vi "_BlankServer.vi"() -> ()   [LabVIEW 2012]
uses:
  <userlib>/ROSforLV/ROS/Code/SubVIs/_ROSControl.ctl
  <userlib>/ROSforLV/ROS/Code/SubVIs/_ROSDirection.ctl
  <userlib>/ROSforLV/ROS/Code/Console/Servers/ServerSubs/ROSLog.ctl
  <userlib>/ROSforLV/ROS/Code/Console/Servers/ServerSubs/MyState.ctl
  <userlib>/ROSforLV/ROS/Code/Console/Servers/ServerSubs/requestTopic.ctl
panel:
  out "Log of port":string
  out "Queue log":string
  out "Last Reply":string
  out "Registered topics":T1[](array[typedef])
  out "Registering":bool
  out "MyState":T3
  out "Setup":string
  out "Cmd Log":T4[](array[typedef])
  out "Connections":T5(array[cluster])
  in  "stop":bool
  in  "ROS":T1={"topic port"=1236, "Node"="/labview", "topic"="/robot/head/command_head_nod", "type"="std_msgs/Bool", "node port"=7000, "error "={"status"=FALSE, "code"=0, "source"=""}, "Direction"=enum."Publisher", "APIs"=[], "Update (ms)"=1, "write queue"=1}
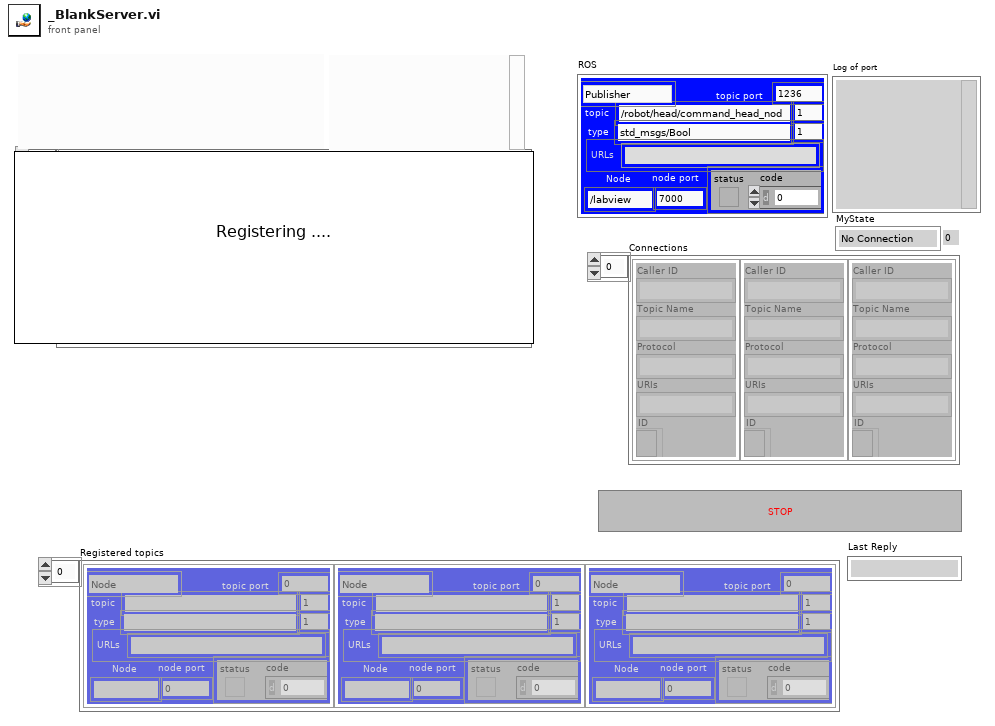
[diagram p1: front panel]
types:
  T1 = typedef "_ROSControl.ctl" = cluster{"topic port":u16, "Node":string, "topic":string, "type":string, "node port":u32, "error ":errorcluster, "Direction":T2, "APIs":string[], "Update (ms)":u16, "write queue":u16}
  T2 = typedef "_ROSDirection.ctl" = enum16{"Node", "Publisher", "Subscriber", "Service Client"}
  T3 = typedef "MyState.ctl" = enum16{"No Connection", "Registered", "Connected", "Close"}
  T4 = typedef "ROSLog.ctl" = cluster{"Sent":string, "Reply":string, "MethodName":string, "success":bool, "Dir1":string, "Dir2":string, "Time Stamp":string, "error":errorcluster, "Preamble":string}
  T5 = cluster{"Caller ID":string, "Topic Name":string, "Protocol":string, "URIs":string, "ID":refnum<k5>}[]
  T6 = enum16{"Reset Log", "Add Client", "Remove Client", "Add Task"}
  T7 = typedef "requestTopic.ctl" = cluster{"New Subscriber":cluster{"Caller ID":string, "Topic Name":string, "Protocol":string, "URIs":string, "ID":refnum<k5>}, "ROS of Server":T1, "new port":u16}
  T8 = cluster{"Code":i32, "Status Message":string, "APIs":string[]}
  T9 = cluster{"Caller ID":string, "Topic Name":string, "Protocol":string, "URIs":string, "ID":refnum<k5>}
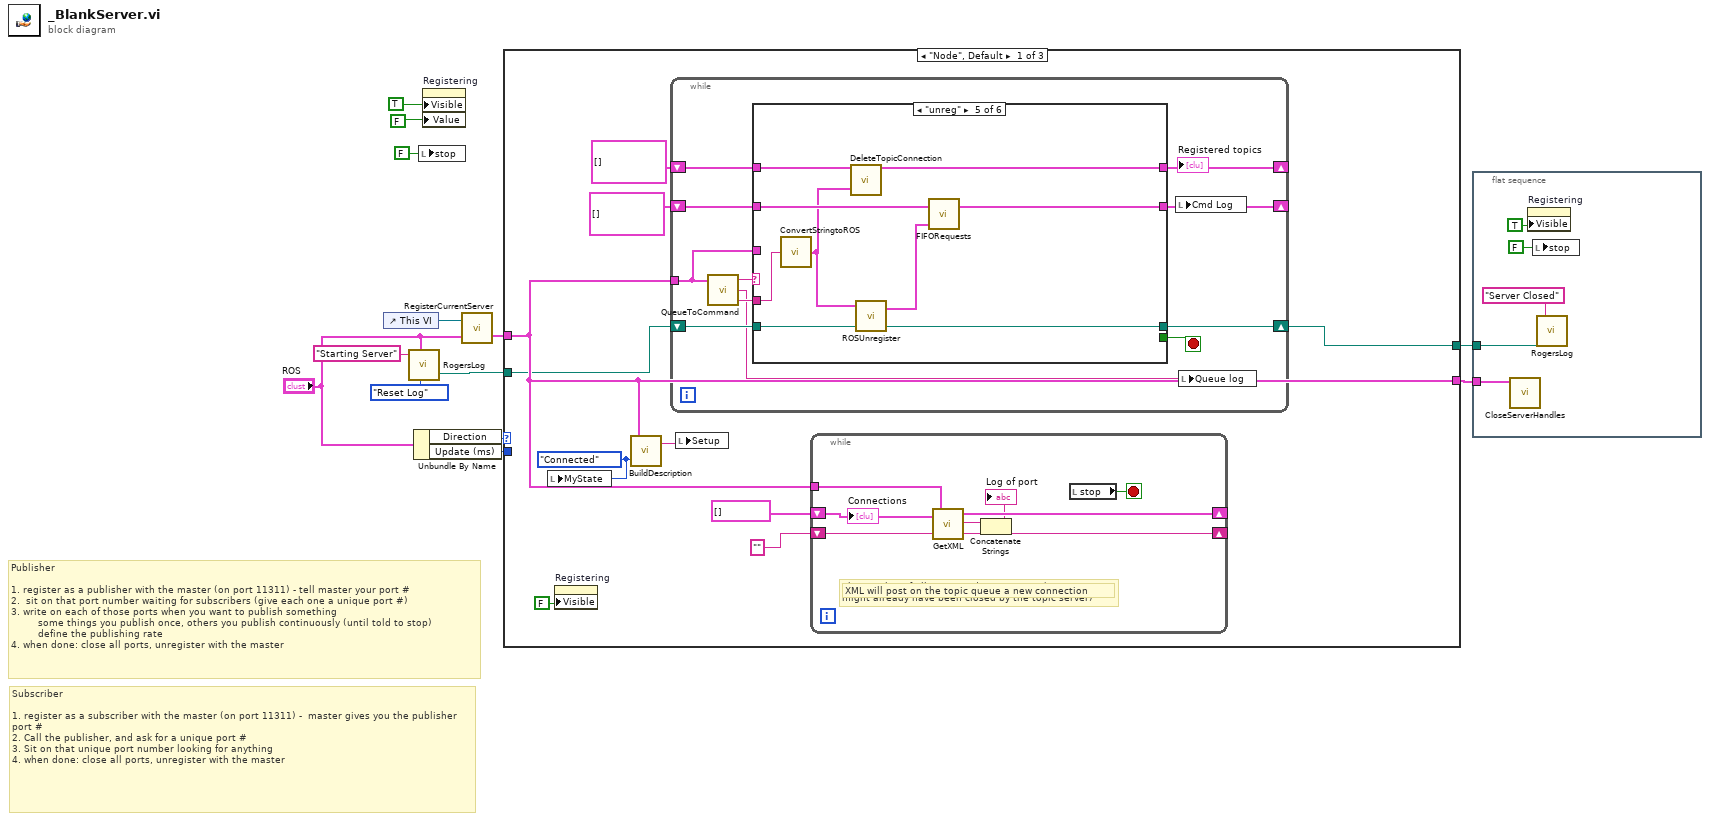
[diagram p0: block diagram]
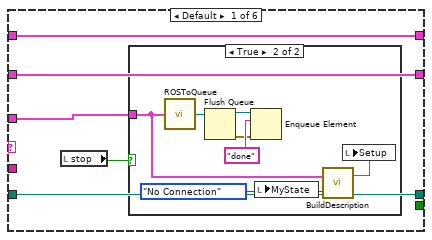
[diagram p2: hidden frame]
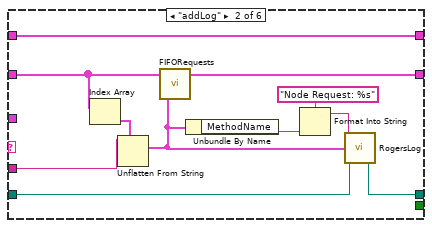
[diagram p4: hidden frame]
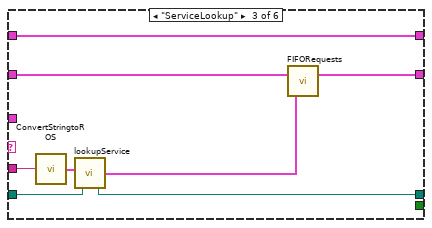
[diagram p5: hidden frame]
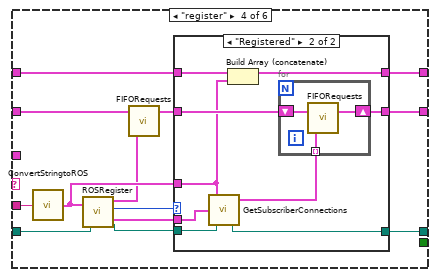
[diagram p6: hidden frame]
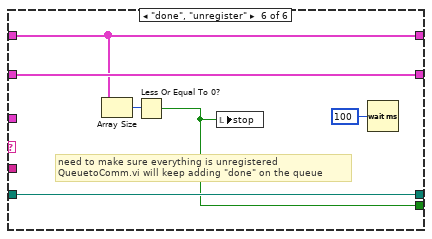
[diagram p8: hidden frame]
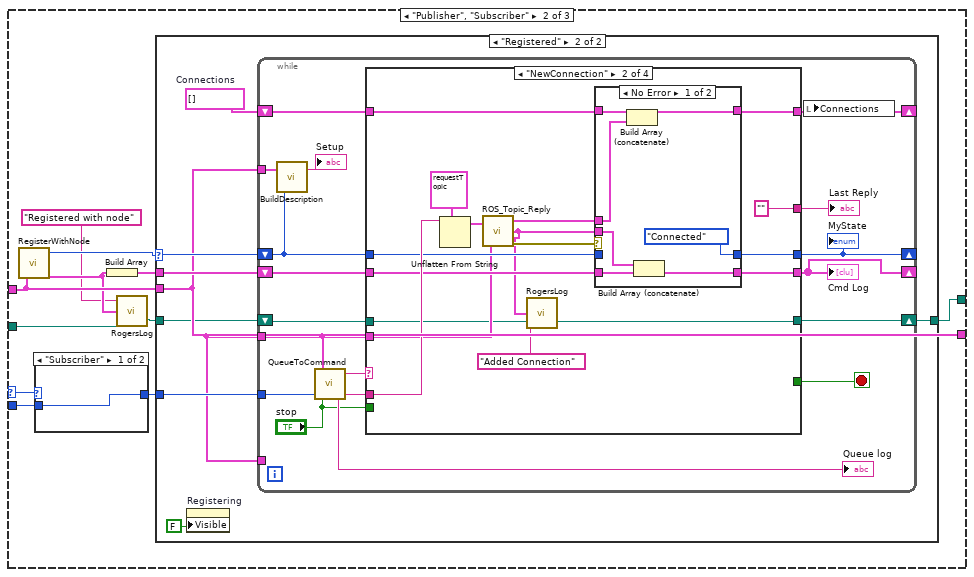
[diagram p9: hidden frame]
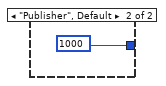
[diagram p10: hidden frame]
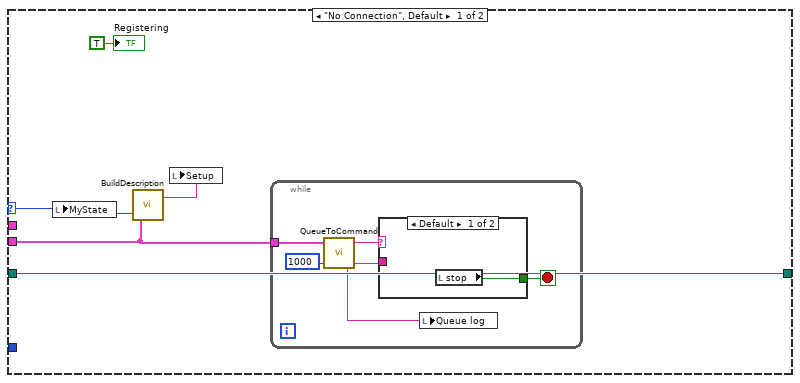
[diagram p11: hidden frame]
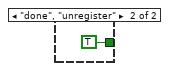
[diagram p12: hidden frame]
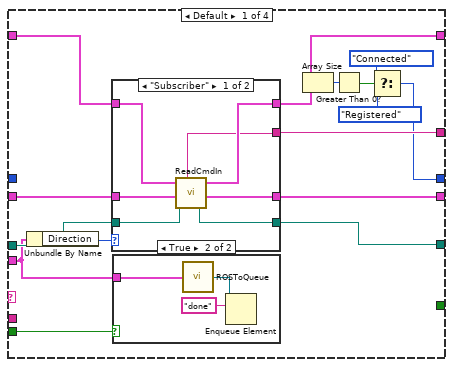
[diagram p13: hidden frame]
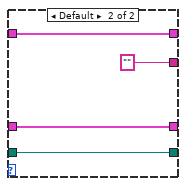
[diagram p14: hidden frame]
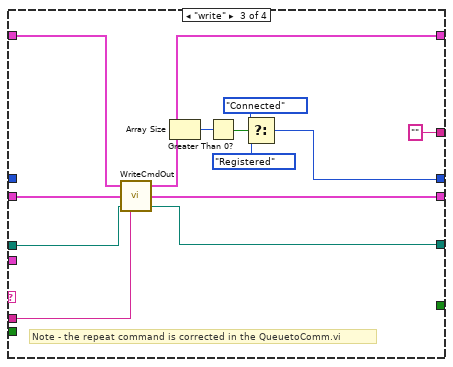
[diagram p17: hidden frame]
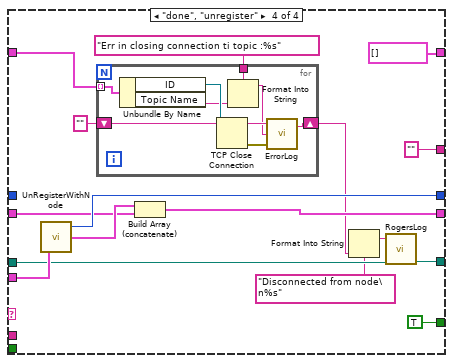
[diagram p18: hidden frame]
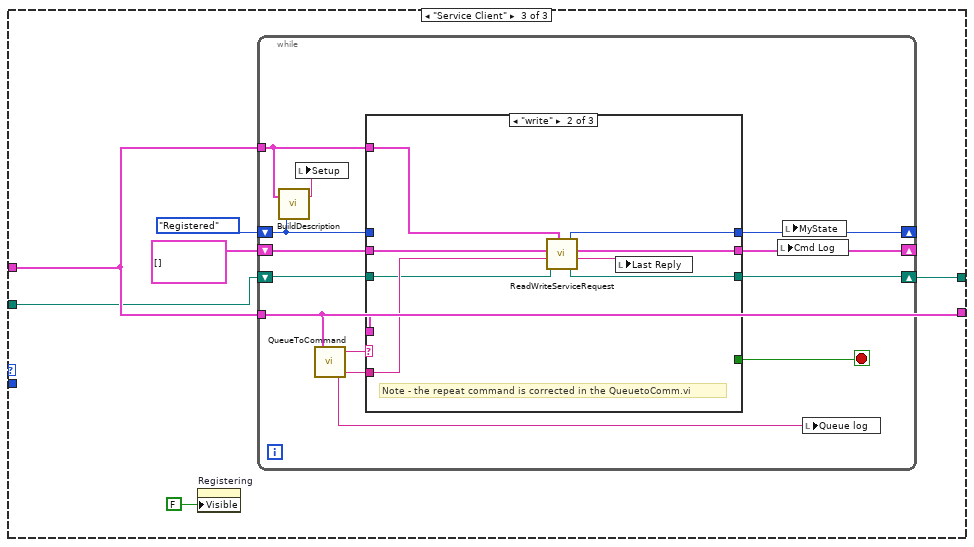
[diagram p19: hidden frame]
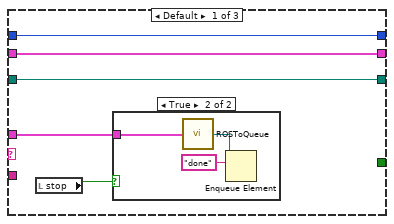
[diagram p20: hidden frame]
diagram:
  # "Subscriber\n\n1. register as a subscriber with the master (on port 11311) -  master gives you the publisher port #\n2. Call the publisher, and ask for a unique port #\n3. Sit on that unique port number looking for anything\n4. when done: close all ports, unregister with the master"
  # "Publisher\n\n1. register as a publisher with the master (on port 11311) - tell master your port #\n2.  sit on that port number waiting for subscribers (give each one a unique port #)\n3. write on each of those ports when you want to publish something\n         some things you publish once, others you publish continuously (until told to stop)\n         define the publishing rate\n4. when done: close all ports, unregister with the master"
  n1 = control-ref of="This VI"() -> (w8:refnum<vi>)
  n2 = call <userlib>:"RogersLog.vi"("Text to add"="Starting Server", "ROS"="ROS", "Task"=T6."Reset Log") -> ("LogPath out"=w2:path)  [unwired: 2 in, 1 out]
  n3 = Unbundle By Name("ROS") -> ("Direction"=w11:T2, "Update (ms)"=w6:u16)
  n4 = local write "stop"(FALSE ("stop")) -> ()
  n5 = property on="Registering" class="Bool (strict)"("Visible"=TRUE ("Registering"), "Value"=FALSE ("Registering")) -> ()  [unwired: 2 in, 2 out]
  n6 = call <userlib>:"RegisterCurrentServer.vi"("ROS in"="ROS", "This VI"=w8) -> ("ROS out"=w7:T1)  [unwired: 1 in]
  n7 = case shown="\"Node\", Default" w11 {
    selector: w11 -> [_ w124 _]
    tunnel: w7 -> [w18 w126 w266]
    tunnel: [w18 w126 w266] -> w9
    tunnel: w6 -> [_ w121 _]
    tunnel: w2 -> [w15 w120 w262]
    tunnel: [w14 w118 w261] -> w1
    frame "Node", Default {
      w21 = MyState."Connected" ("MyState")
      n8 = local write "MyState"(w21) -> ()
      n9 = property on="Registering" class="Bool (strict)"("Visible"=FALSE ("Registering")) -> ()  [unwired: 2 in, 2 out]
      n10 = call <userlib>:"BuildDescription.vi"("MyState"=w21, "ROS in"=w18) -> ("Setup"=w22:string)  [unwired: 1 in]
      n11 = while {
        shift-right: [w25] -> w14
        shift-left: w15 -> [w33]
        shift-right: [w26] -> _
        shift-left: T4[] [] ("Requests Out") -> [w32]
        shift-right: [w31] -> _
        shift-left: T1[] [] -> [w30]
        tunnel: w18 -> [w24]
        stop <- w34 stop-if-true
        n12 = call <userlib>:"QueueToCommand.vi"("ROS"=w24) -> ("data"=w28:string, "Queue log"=w27:string, "Command"=w29:string)  [unwired: 2 in]
        n13 = case shown="\"unreg\"" w29 {
          tunnel: [_ _ _ _ _ w104] -> w34
          tunnel: w28 -> [_ w56 w64 w78 w102 _]
          tunnel: w33 -> [w39 w48 w59 w77 w101 w108]
          tunnel: [w39 w47 w58 w66 w100 w108] -> w25
          tunnel: [w38 w53 w60 w76 w98 w107] -> w26
          tunnel: w32 -> [w38 w54 w61 w69 w99 w107]
          tunnel: [w37 w57 w65 w74 w95 w106] -> w31
          tunnel: w30 -> [w37 w57 w65 w75 w96 w106]
          tunnel: w24 -> [w35 _ _ _ _ _]
          frame Default {
            n14 = local read "stop"() -> (w36:bool)
            n15 = case shown="True" w36 {
              tunnel: w35 -> [_ w41]
              frame False {
              }
              frame True {
                w42 = MyState."No Connection" ("MyState")
                n16 = call <userlib>:"ROSToQueue.vi"("ROS"=w41) -> ("queue"=w44:refnum<queue>)  [unwired: 3 in, 1 out]
                n17 = Flush Queue(queue=w44) -> (queue out=w40:refnum<queue>, error out=w45:errorcluster)  [unwired: 1 in, 1 out]
                n18 = Enqueue Element(queue=w40, element="done" ("regular expression"), error in (no error)=w45) -> ()  [unwired: 1 in, 3 out]
                n19 = local write "MyState"(w42) -> ()
                n20 = call <userlib>:"BuildDescription.vi"("MyState"=w42, "ROS in"=w41) -> ("Setup"=w43:string)  [unwired: 1 in]
                n21 = local write "Setup"(w43) -> ()
              }
            }
          }
          frame "addLog" {
            n22 = Index Array(array=w54) -> (element=w55:T4)  [unwired: 1 in]
            n23 = Unflatten From String(type=w55, binary string=w56) -> (value=w51:T4)  [unwired: 3 in, 2 out]
            n24 = call <userlib>:"FIFORequests.vi"("Log"=w51, "Requests in"=w54) -> ("Requests out"=w53:T4[])  [unwired: 1 in]
            n25 = Unbundle By Name(w51) -> ("MethodName"=w50:string)
            n26 = Format Into String(format string="Node Request: %s", w50) -> (resulting string=w49:string)  [unwired: 2 in, 1 out]
            n27 = call <userlib>:"RogersLog.vi"("Text to add"=w49, "Log"=w51, "LogPath in"=w48) -> ("LogPath out"=w47:path)  [unwired: 2 in, 1 out]
          }
          frame "ServiceLookup" {
            n28 = call <userlib>:"ConvertStringtoROS.vi"("string in"=w64) -> ("ROS"=w63:T1)
            n29 = call <userlib>:"lookupService.vi"("Err In"=w59, "Service ROS"=w63) -> ("Err Out"=w58:path, "Log"=w62:T4)  [unwired: 2 in]
            n30 = call <userlib>:"FIFORequests.vi"("Log"=w62, "Requests in"=w61) -> ("Requests out"=w60:T4[])  [unwired: 1 in]
          }
          frame "register" {
            n31 = call <userlib>:"ConvertStringtoROS.vi"("string in"=w78) -> ("ROS"=w73:T1)
            n32 = call <userlib>:"ROSRegister.vi"("Err In"=w77, "ROS to register"=w73) -> ("Err Out"=w67:path, "Response"=w72:T8, "MyState"=w71:T3, "Log"=w70:T4)
            n33 = call <userlib>:"FIFORequests.vi"("Log"=w70, "Requests in"=w69) -> ("Requests out"=w68:T4[])  [unwired: 1 in]
            n34 = case shown="\"Registered\"" w71 {
              tunnel: w68 -> [w80 w90]
              tunnel: [w80 w89] -> w76
              tunnel: w75 -> [w81 w88]
              tunnel: [w81 w87] -> w74
              tunnel: w73 -> [_ w85]
              tunnel: w72 -> [_ w84]
              tunnel: w67 -> [w79 w83]
              tunnel: [w79 w82] -> w66
              frame Default {
              }
              frame "Registered" {
                n35 = call <userlib>:"GetSubscriberConnections.vi"("Err in"=w83, "Response"=w84, "ROS registered"=w85) -> ("Err out"=w82:path, "Logs out"=w86:T4[])  [unwired: 1 out]
                n36 = Build Array (concatenate)(w88, w85) -> (w87:T1[])
                n37 = for {
                  tunnel: w86 -> [w91] mode=indexing
                  shift-right: [w92] -> w89
                  shift-left: w90 -> [w93]
                  n38 = call <userlib>:"FIFORequests.vi"("Log"=w91, "Requests in"=w93) -> ("Requests out"=w92:T4[])  [unwired: 1 in]
                }
              }
            }
          }
          frame "unreg" {
            n39 = call <userlib>:"ConvertStringtoROS.vi"("string in"=w102) -> ("ROS"=w94:T1)
            n40 = call <userlib>:"DeleteTopicConnection.vi"("ROS"=w94, "Con In"=w96) -> ("Con out"=w95:T1[])
            n41 = call <userlib>:"ROSUnregister.vi"("Err in"=w101, "Server ROS"=w94) -> ("Err out"=w100:path, "Log"=w97:T4)  [unwired: 1 in]
            n42 = call <userlib>:"FIFORequests.vi"("Log"=w97, "Requests in"=w99) -> ("Requests out"=w98:T4[])  [unwired: 1 in]
          }
          frame "done", "unregister" {
            # "need to make sure everything is unregistered\nQueuetoComm.vi will keep adding \"done\" on the queue"
            n43 = Array Size(array=w106) -> (size(s)=w105:i32)
            n44 = Less Or Equal To 0?(x=w105) -> (x <= 0?=w104:bool)
            n45 = local write "stop"(w104) -> ()
            n46 = Wait (ms)(milliseconds to wait=u32 100) -> ()  [unwired: 1 out]
          }
        }
        "Registered topics" <- w31
        n47 = local write "Cmd Log"(w26) -> ()
        n48 = local write "Queue log"(w27) -> ()
      }
      n49 = local write "Setup"(w22) -> ()
      n50 = while {
        shift-right: [w115] -> _
        shift-left: T5 [] ("Subscribers") -> [w109]
        tunnel: w18 -> [w114]
        shift-right: [w110] -> _
        shift-left: "" ("String out") -> [w112]
        stop <- w113 stop-if-true
        # "This is a log of all requested connections (some\nmight already have been closed by the topic server)"
        # "XML will post on the topic queue a new connection"
        n51 = call <userlib>:"GetXML.vi"("Node ROS"=w114, "Subscribers in"=w109) -> ("reply"=w111:string, "Subscribers Out"=w115:T5)  [unwired: 1 in]
        n52 = Concatenate Strings(w111, w112) -> (w110:string)
        "Log of port" <- w110
        n53 = local read "stop"() -> (w113:bool)
        "Connections" <- w109
      }
    }
    frame "Publisher", "Subscriber" {
      n54 = call <userlib>:"RegisterWithNode.vi"("ROS"=w126) -> ("MyState"=w125:T3, "Log"=w117:T4)  [unwired: 1 in]
      n55 = case shown="\"Subscriber\"" w124 {
        tunnel: [w127 1000 ("timeout in ms (1000)")] -> w123
        tunnel: w121 -> [w127 _]
        frame "Subscriber" {
        }
        frame "Publisher", Default {
        }
      }
      n56 = Build Array(w117) -> (w122:T4[])
      n57 = call <userlib>:"RogersLog.vi"("Text to add"="Registered with node" ("format string"), "Log"=w117, "LogPath in"=w120) -> ("LogPath out"=w119:path)  [unwired: 2 in, 1 out]
      n58 = case shown="\"Registered\"" w125 {
        selector: w125 -> [w132 w148]
        tunnel: w126 -> [w130 w143]
        tunnel: w123 -> [_ w146]
        tunnel: w122 -> [_ w145]
        tunnel: w119 -> [w129 w144]
        tunnel: [w129 w142] -> w118
        frame "No Connection", Default {
          n59 = local write "MyState"(w132) -> ()
          n60 = call <userlib>:"BuildDescription.vi"("MyState"=w132, "ROS in"=w130) -> ("Setup"=w133:string)  [unwired: 1 in]
          n61 = local write "Setup"(w133) -> ()
          n62 = while {
            tunnel: w130 -> [w134]
            stop <- w139 stop-if-true
            n63 = call <userlib>:"QueueToCommand.vi"("timeout"=1000 ("timeout in ms (-1)"), "ROS"=w134) -> ("data"=w138:string, "Queue log"=w135:string, "Command"=w136:string)  [unwired: 1 in]
            n64 = case shown="Default" w136 {
              tunnel: [w140 TRUE] -> w139
              tunnel: w138 -> [_ _]
              frame Default {
                n65 = local read "stop"() -> (w140:bool)
              }
              frame "done", "unregister" {
              }
            }
            n66 = local write "Queue log"(w135) -> ()
          }
          "Registering" <- TRUE ("Registering")
        }
        frame "Registered" {
          w149 = T5 []  # Connections
          n67 = property on="Registering" class="Bool (strict)"("Visible"=FALSE ("Registering")) -> ()  [unwired: 2 in, 2 out]
          n68 = while {
            shift-right: [w150] -> w142
            shift-left: w144 -> [w167]
            shift-right: [w164] -> _
            shift-left: w145 -> [w165]
            shift-right: [w162] -> _
            shift-left: w148 -> [w153]
            tunnel: w143 -> [w161]
            tunnel: w143 -> [w152]
            shift-right: [w155] -> _
            shift-left: w149 -> [w160]
            tunnel: w146 -> [w154]
            tunnel: w143 -> [_]
            stop <- w159 stop-if-true
            n69 = call <userlib>:"BuildDescription.vi"("MyState"=w153, "ROS in"=w161) -> ("Setup"=→"Setup":string)  [unwired: 1 in]
            n70 = call <userlib>:"QueueToCommand.vi"("timeout"=w154, "Stop Btn Pressed?"="stop", "ROS"=w152) -> ("data"=w166:string, "Queue log"=→"Queue log":string, "Command"=w157:string)
            n71 = case shown="\"NewConnection\"" w157 {
              tunnel: [w180 w197 w236 w241] -> w150
              tunnel: w167 -> [w179 w200 w224 w242]
              tunnel: [w171 w204 w227 w252] -> w162
              tunnel: w166 -> [_ w209 w233 _]
              tunnel: w165 -> [w178 w208 w235 w248]
              tunnel: [w181 w207 w234 w247] -> w164
              tunnel: w160 -> [w177 w213 w231 w246]
              tunnel: [w172 w212 w225 T5 [] ("Connections Out")] -> w155
              tunnel: [_ _ _ TRUE] -> w159
              tunnel: [w182 "" ("String out") "" ("String out") "" ("String out")] -> w158
              tunnel: w153 -> [_ w203 _ _]
              tunnel: w152 -> [w169 w201 _ w244]
              tunnel: "stop" -> [w168 _ _ _]
              frame Default {
                n72 = Unbundle By Name(w169) -> ("Direction"=w170:T2)
                n73 = case shown="\"Subscriber\"" w170 {
                  tunnel: [w185 "" ("String out")] -> w182
                  tunnel: [w189 w191] -> w172
                  tunnel: [w188 w192] -> w181
                  tunnel: [w187 w190] -> w180
                  tunnel: w179 -> [w183 w190]
                  tunnel: w178 -> [w186 w192]
                  tunnel: w177 -> [w184 w191]
                  frame "Subscriber" {
                    n74 = call <userlib>:"ReadCmdIn.vi"("Connections"=w184, "Log in"=w186, "Err in"=w183) -> ("data"=w185:string, "Connections out"=w189:T5, "Log out"=w188:T4[], "Err out"=w187:path)  [unwired: 1 in]
                  }
                  frame Default {
                  }
                }
                n75 = case shown="True" w168 {
                  tunnel: w169 -> [_ w194]
                  frame False {
                  }
                  frame True {
                    n76 = call <userlib>:"ROSToQueue.vi"("ROS"=w194) -> ("queue"=w195:refnum<queue>)  [unwired: 3 in, 1 out]
                    n77 = Enqueue Element(queue=w195, element="done") -> ()  [unwired: 2 in, 3 out]
                  }
                }
                n78 = Array Size(array=w172) -> (size(s)=w176:i32)
                n79 = Greater Than 0?(x=w176) -> (x > 0?=w173:bool)
                n80 = Select(t=MyState."Connected" ("f"), s=w173, f=MyState."Registered") -> (s? t:f=w171:T3)
              }
              frame "NewConnection" {
                n81 = Unflatten From String(type=T7 {"New Subscriber"={"Caller ID"="", "Topic Name"="", "Protocol"="", "URIs"="", "ID"=refnum}, "ROS of Server"={"topic port"=0, "Node"="", "topic"="", "type"="", "node port"=0, "error "={"status"=FALSE, "code"=0, "source"=""}, "Direction"=enum."Node", "APIs"=[], "Update (ms)"=0, "write queue"=0}, "new port"=0} ("data"), binary string=w209) -> (value=w206:T7)  [unwired: 3 in, 2 out]
                n82 = call <userlib>:"ROS_Topic_Reply.vi"("data"=w206, "My ROS"=w201) -> ("Subscriber out"=w210:T9, "Log"=w199:T4, "error IO"=w205:errorcluster)
                n83 = call <userlib>:"RogersLog.vi"("Text to add"="Added Connection", "Log"=w199, "LogPath in"=w200) -> ("LogPath out"=w197:path)  [unwired: 2 in, 1 out]
                n84 = case shown="No Error" w205 {
                  tunnel: w213 -> [w220 w223]
                  tunnel: [w219 w223] -> w212
                  tunnel: w210 -> [w218 _]
                  tunnel: w199 -> [w217 _]
                  tunnel: w208 -> [w216 w222]
                  tunnel: [w215 w222] -> w207
                  tunnel: [MyState."Connected" ("MyState") w221] -> w204
                  tunnel: w203 -> [_ w221]
                  frame No Error {
                    n85 = Build Array (concatenate)(w220, w218) -> (w219:T5)
                    n86 = Build Array (concatenate)(w217, w216) -> (w215:T4[])
                  }
                  frame Error {
                  }
                }
              }
              frame "write" {
                # "Note - the repeat command is corrected in the QueuetoComm.vi"
                n87 = call <userlib>:"WriteCmdOut.vi"("Connections In"=w231, "Log in"=w235, "Err in"=w224, "data"=w233) -> ("Connections Out"=w225:T5, "Log out"=w234:T4[], "Err out"=w236:path)  [unwired: 1 in]
                n88 = Array Size(array=w225) -> (size(s)=w226:i32)
                n89 = Greater Than 0?(x=w226) -> (x > 0?=w230:bool)
                n90 = Select(t=MyState."Connected" ("f"), s=w230, f=MyState."Registered") -> (s? t:f=w227:T3)
              }
              frame "done", "unregister" {
                n91 = call <userlib>:"UnRegisterWithNode.vi"("ROS"=w244) -> ("MyState"=w252:T3, "Log"=w249:T4)  [unwired: 2 in]
                n92 = for {
                  tunnel: w246 -> [w260] mode=indexing
                  shift-right: [w258] -> w239
                  shift-left: "" ("String out") -> [w257]
                  tunnel: "Err in closing connection ti topic :%s" ("String in") -> [w255]
                  n93 = Unbundle By Name(w260) -> ("ID"=w259:refnum<k5>, "Topic Name"=w254:string)
                  n94 = TCP Close Connection(connection ID=w259) -> (error out=w256:errorcluster)  [unwired: 2 in, 1 out]
                  n95 = Format Into String(format string=w255, w254) -> (resulting string=w253:string)  [unwired: 2 in, 1 out]
                  n96 = call <userlib>:"ErrorLog.vi"("error in"=w256, "String in"=w253, "Error String"=w257) -> ("String out"=w258:string)  [unwired: 1 out]
                }
                n97 = Build Array (concatenate)(w249, w248) -> (w247:T4[])
                n98 = Format Into String(format string="Disconnected from node\n%s", w239) -> (resulting string=w238:string)  [unwired: 2 in, 1 out]
                n99 = call <userlib>:"RogersLog.vi"("Text to add"=w238, "LogPath in"=w242) -> ("LogPath out"=w241:path)  [unwired: 3 in, 1 out]
              }
            }
            "Cmd Log" <- w164
            "MyState" <- w162
            "Last Reply" <- w158
            n100 = local write "Connections"(w155) -> ()
          }
        }
      }
    }
    frame "Service Client" {
      n101 = property on="Registering" class="Bool (strict)"("Visible"=FALSE ("Registering")) -> ()  [unwired: 2 in, 2 out]
      n102 = while {
        shift-right: [w267] -> w261
        shift-left: w262 -> [w279]
        shift-right: [w269] -> _
        shift-left: T4[] [] ("Log") -> [w277]
        shift-right: [w273] -> _
        shift-left: MyState."Registered" ("MyState") -> [w276]
        tunnel: w266 -> [w270]
        tunnel: w266 -> [w268]
        stop <- w275 stop-if-true
        n103 = call <userlib>:"BuildDescription.vi"("MyState"=w276, "ROS in"=w270) -> ("Setup"=w271:string)  [unwired: 1 in]
        n104 = local write "Setup"(w271) -> ()
        n105 = call <userlib>:"QueueToCommand.vi"("ROS"=w268) -> ("data"=w278:string, "Queue log"=w272:string, "Command"=w274:string)  [unwired: 2 in]
        n106 = case shown="\"write\"" w274 {
          tunnel: [w281 w289 w298] -> w267
          tunnel: w279 -> [w281 w290 w298]
          tunnel: [w283 w293 MyState."No Connection" ("MyState")] -> w273
          tunnel: w278 -> [_ w291 _]
          tunnel: w277 -> [w282 w295 w299]
          tunnel: [w282 w294 w299] -> w269
          tunnel: w276 -> [w283 _ _]
          tunnel: [_ _ TRUE] -> w275
          tunnel: w270 -> [_ w292 _]
          tunnel: w268 -> [w280 _ _]
          frame Default {
            n107 = local read "stop"() -> (w284:bool)
            n108 = case shown="True" w284 {
              tunnel: w280 -> [_ w285]
              frame False {
              }
              frame True {
                n109 = call <userlib>:"ROSToQueue.vi"("ROS"=w285) -> ("queue"=w286:refnum<queue>)  [unwired: 3 in, 1 out]
                n110 = Enqueue Element(queue=w286, element="done") -> ()  [unwired: 2 in, 3 out]
              }
            }
          }
          frame "write" {
            # "Note - the repeat command is corrected in the QueuetoComm.vi"
            n111 = call <userlib>:"ReadWriteServiceRequest.vi"("Service ROS"=w292, "Error in"=w290, "data"=w291, "Log in"=w295) -> ("Error out"=w289:path, "String Read"=w288:string, "Log"=w294:T4[], "MyState"=w293:T3)  [unwired: 1 in]
            n112 = local write "Last Reply"(w288) -> ()
          }
          frame "done", "unregister" {
            # "stop all repeating connections"
          }
        }
        n113 = local write "Cmd Log"(w269) -> ()
        n114 = local write "MyState"(w273) -> ()
        n115 = local write "Queue log"(w272) -> ()
      }
    }
  }
  n116 = flat-sequence {
    tunnel: w9 -> [w302]
    tunnel: w1 -> [w301]
    frame #0 {
      n117 = call <userlib>:"CloseServerHandles.vi"("ROS"=w302) -> ()
      n118 = property on="Registering" class="Bool (strict)"("Visible"=TRUE ("Registering")) -> ()  [unwired: 2 in, 2 out]
      n119 = local write "stop"(FALSE ("stop")) -> ()
      n120 = call <userlib>:"RogersLog.vi"("Text to add"="Server Closed", "LogPath in"=w301) -> ()  [unwired: 3 in, 2 out]
    }
  }
